vi "RenderRobotPose.vi"(0 "Robot X (in)":dbl, 1 "Robot Width (in)":dbl=30.0 format="%#_13g", 2 "Robot Length (in)":dbl=30.0 format="%#_13g", 3 "Buffer Time (min)":dbl=5.0 format="%#_13g", 5 "Robot Y (in)":dbl, 7 "Targeting Predictions":dbl[](array[numeric])=[0.0, 0.0, 0.0, 0.0], 9 "Robot Heading (deg)":dbl, 11 "Turret Heading (deg)":dbl, 12 "Robot Enabled":bool, 14 "Reset":bool) -> (6 "Robot Pose":cluster{dbl[], dbl[]}[](graph))   [LabVIEW 2020]
doc: "This VI takes the robot pose information as input and renders a plot to display it. At this time, only square robot dimensions are supported."
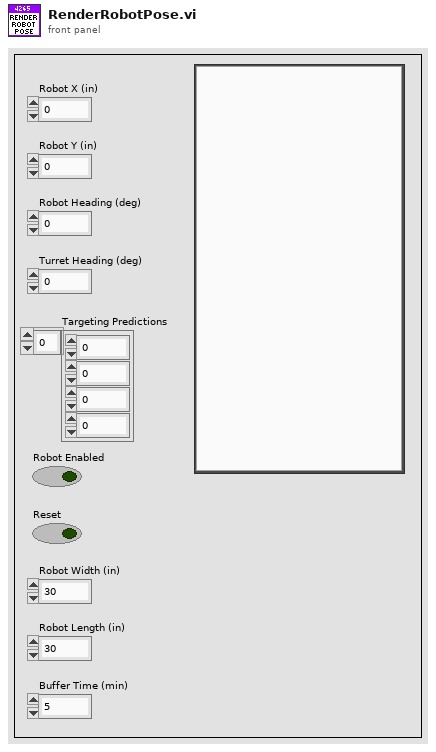
[diagram p1: front panel]
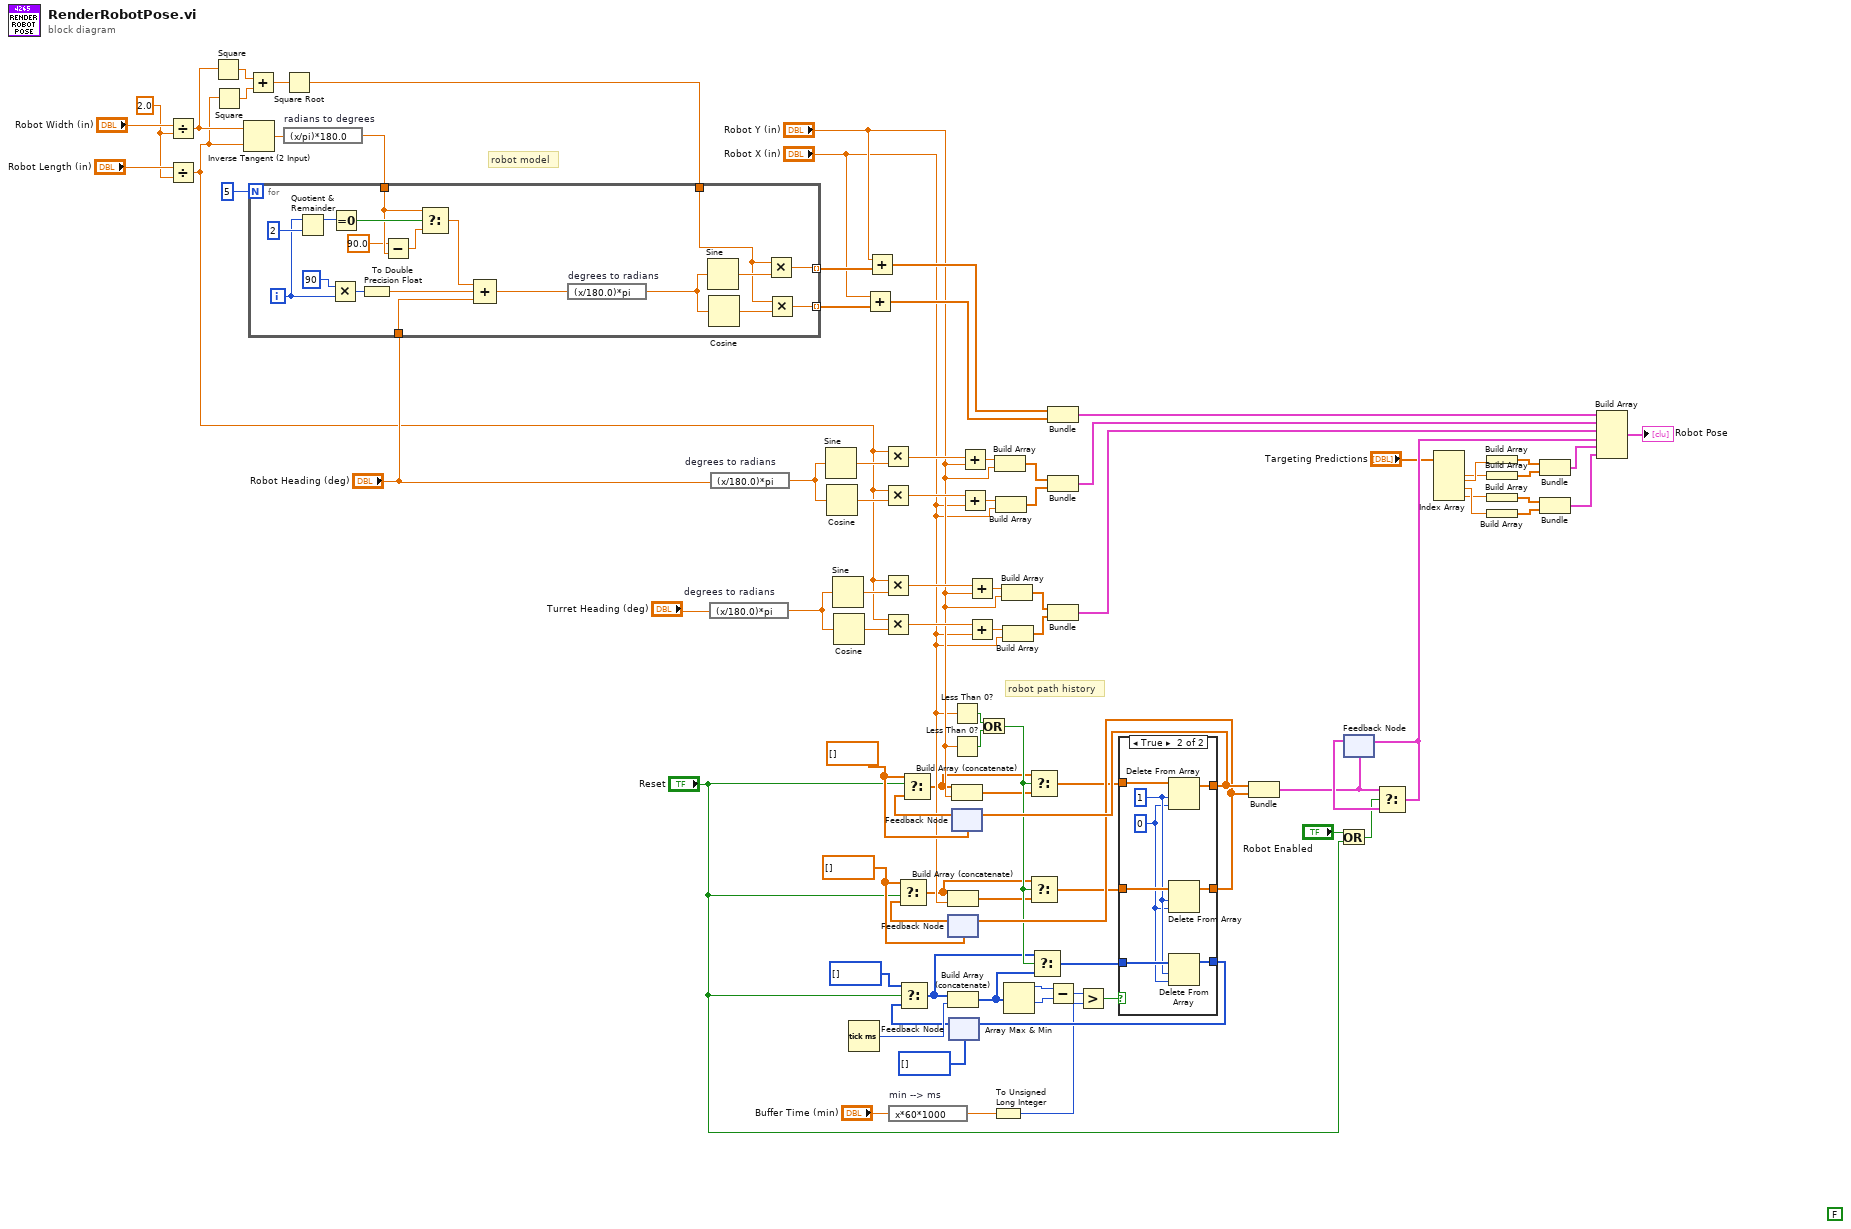
[diagram p0: block diagram]
diagram:
  w20 = 2.0
  (unwired) FALSE
  w39 = dbl[] [] ("t")
  w38 = dbl[] [] ("t")
  # "robot model"
  # "robot path history"
  n1 = Divide(x="Robot Width (in)", y=w20) -> (x/y=w17:dbl)
  n2 = Divide(x="Robot Length (in)", y=w20) -> (x/y=w16:dbl)
  n3 = Square(x=w17) -> (x^2=w14:dbl)
  n4 = Square(x=w16) -> (x^2=w15:dbl)
  n5 = Inverse Tangent (2 Input)(1:w16, 2:w17) -> (0:w19:dbl)
  n6 = Add(x=w14, y=w15) -> (x+y=w13:dbl)
  n7 = Square Root(x=w13) -> (sqrt(x)=w12:dbl)
  n8 = expression code="(x/pi)*180.0" "radians to degrees"(w19) -> (w18:dbl)
  n9 = for {
    N: 5 -> [_]
    tunnel: [w105] -> w88 mode=indexing
    tunnel: [w104] -> w87 mode=indexing
    tunnel: "Robot Heading (deg)" -> [w99]
    tunnel: w18 -> [w95]
    tunnel: w12 -> [w90]
    i -> [w91]
    n10 = Quotient & Remainder(x=w91, y=2) -> (x-y*floor(x/y)=w97:i32)  [unwired: 1 out]
    n11 = Multiply(x=90, y=w91) -> (x*y=w102:i32)
    n12 = Equal To 0?(x=w97) -> (x = 0?=w96:bool)
    n13 = To Double Precision Float(number=w102) -> (double precision float=w101:dbl)
    n14 = Subtract(x=90.0, y=w95) -> (x-y=w94:dbl)
    n15 = Select(t=w95, s=w96, f=w94) -> (s? t:f=w92:dbl)
    n16 = Compound Arithmetic op=ADD(w92, w101, w99) -> (w100:dbl)
    n17 = expression code="(x/180.0)*pi" "degrees to radians"(w100) -> (w107:dbl)
    n18 = Sine(x=w107) -> (sin(x)=w106:dbl)
    n19 = Cosine(x=w107) -> (cos(x)=w108:dbl)
    n20 = Multiply(x=w90, y=w106) -> (x*y=w104:dbl)
    n21 = Multiply(x=w90, y=w108) -> (x*y=w105:dbl)
  }
  n22 = expression code="(x/180.0)*pi" "degrees to radians"("Turret Heading (deg)") -> (w64:dbl)
  n23 = expression code="(x/180.0)*pi" "degrees to radians"("Robot Heading (deg)") -> (w53:dbl)
  n24 = Sine(x=w53) -> (sin(x)=w52:dbl)
  n25 = Cosine(x=w53) -> (cos(x)=w51:dbl)
  n26 = Sine(x=w64) -> (sin(x)=w63:dbl)
  n27 = Cosine(x=w64) -> (cos(x)=w62:dbl)
  n28 = Tick Count (ms)() -> (millisecond timer value=w71:u32)
  n29 = Add(x="Robot X (in)", y=w88) -> (x+y=w85:dbl[])
  n30 = Add(x="Robot Y (in)", y=w87) -> (x+y=w84:dbl[])
  n31 = Multiply(x=w16, y=w52) -> (x*y=w50:dbl)
  n32 = Multiply(x=w16, y=w51) -> (x*y=w49:dbl)
  n33 = Multiply(x=w16, y=w63) -> (x*y=w61:dbl)
  n34 = Multiply(x=w16, y=w62) -> (x*y=w60:dbl)
  n35 = expression code="x*60*1000" "min --> ms"("Buffer Time (min)") -> (w76:dbl)
  n36 = feedback #1(w38) -> (w67:dbl[])
  n37 = Select(t=w38, s="Reset", f=w67) -> (s? t:f=w27:dbl[])
  n38 = Build Array (concatenate)(w27, "Robot X (in)") -> (w28:dbl[])
  n39 = feedback #2(u32[] []) -> (w69:u32[])
  n40 = Select(t=u32[] [], s="Reset", f=w69) -> (s? t:f=w32:u32[])
  n41 = Build Array (concatenate)(w32, w71) -> (w31:u32[])
  n42 = Less Than 0?(x="Robot X (in)") -> (x < 0?=w35:bool)
  n43 = Less Than 0?(x="Robot Y (in)") -> (x < 0?=w36:bool)
  n44 = feedback #3(w39) -> (w70:dbl[])
  n45 = Select(t=w39, s="Reset", f=w70) -> (s? t:f=w29:dbl[])
  n46 = Build Array (concatenate)(w29, "Robot Y (in)") -> (w30:dbl[])
  n47 = Add(x=w50, y="Robot Y (in)") -> (x+y=w48:dbl)
  n48 = Add(x=w49, y="Robot X (in)") -> (x+y=w47:dbl)
  n49 = Add(x=w61, y="Robot Y (in)") -> (x+y=w59:dbl)
  n50 = Add(x=w60, y="Robot X (in)") -> (x+y=w58:dbl)
  n51 = Or(x=w35, y=w36) -> (x .or. y?=w34:bool)
  n52 = To Unsigned Long Integer(number=w76) -> (unsigned 32bit integer=w77:u32)
  n53 = Build Array(w48, "Robot Y (in)") -> (w46:dbl[])
  n54 = Build Array(w47, "Robot X (in)") -> (w45:dbl[])
  n55 = Build Array(w59, "Robot Y (in)") -> (w57:dbl[])
  n56 = Build Array(w58, "Robot X (in)") -> (w56:dbl[])
  n57 = Array Max & Min(array=w31) -> (max value=w73:u32, min value=w74:u32)  [unwired: 2 out]
  n58 = Select(t=w29, s=w34, f=w30) -> (s? t:f=w41:dbl[])
  n59 = Select(t=w27, s=w34, f=w28) -> (s? t:f=w40:dbl[])
  n60 = Select(t=w32, s=w34, f=w31) -> (s? t:f=w33:u32[])
  n61 = Bundle(w84, w85) -> (w55:cluster{dbl[], dbl[]})  [unwired: 1 in]
  n62 = Bundle(w46, w45) -> (w54:cluster{dbl[], dbl[]})  [unwired: 1 in]
  n63 = Bundle(w57, w56) -> (w65:cluster{dbl[], dbl[]})  [unwired: 1 in]
  n64 = Subtract(x=w73, y=w74) -> (x-y=w75:u32)
  n65 = Greater?(x=w75, y=w77) -> (0:w79:bool)
  n66 = case shown="True" w79 {
    tunnel: w33 -> [w109 w117]
    tunnel: w40 -> [w110 w118]
    tunnel: w41 -> [w111 w119]
    tunnel: [w111 w114] -> w82
    tunnel: [w110 w113] -> w81
    tunnel: [w109 w112] -> w80
    frame False {
    }
    frame True {
      w115 = 0 ("index")
      w116 = 1 ("length")
      n67 = Delete From Array(array=w119, length=w116, index=w115) -> (array with subset deleted=w114:dbl[])  [unwired: 1 out]
      n68 = Delete From Array(array=w118, length=w116, index=w115) -> (array with subset deleted=w113:dbl[])  [unwired: 1 out]
      n69 = Delete From Array(array=w117, length=w116, index=w115) -> (array with subset deleted=w112:u32[])  [unwired: 1 out]
    }
  }
  n70 = feedback-in #1(w81) -> ()
  n71 = feedback-in #2(w80) -> ()
  n72 = feedback-in #3(w82) -> ()
  n73 = Bundle("t"=w82, "t"=w81) -> (w44:cluster{"t":dbl[], "t":dbl[]})  [unwired: 1 in]
  n74 = Or(x="Robot Enabled", y="Reset") -> (x .or. y?=w24:bool)
  n75 = feedback #4(w44) -> (w83:cluster{"t":dbl[], "t":dbl[]})
  n76 = Select(t=w44, s=w24, f=w83) -> (s? t:f=w43:cluster{"t":dbl[], "t":dbl[]})
  n77 = feedback-in #4(w43) -> ()
  n78 = Index Array(array="Targeting Predictions") -> (element #1=w3:dbl, element #2=w4:dbl, element #3=w2:dbl, element #4=w1:dbl)  [unwired: 4 in]
  n79 = Build Array(w4) -> (w11:dbl[])
  n80 = Build Array(w3) -> (w10:dbl[])
  n81 = Build Array(w1) -> (w9:dbl[])
  n82 = Build Array(w2) -> (w8:dbl[])
  n83 = Bundle(w11, w10) -> (w6:cluster{dbl[], dbl[]})  [unwired: 1 in]
  n84 = Bundle(w9, w8) -> (w7:cluster{dbl[], dbl[]})  [unwired: 1 in]
  n85 = Build Array(w55, w54, w65, w43, w6, w7) -> (→"Robot Pose":cluster{"t":dbl[], "t":dbl[]}[])
